vi "Measurement Loop.vi"(7 "measure call context in":refnum<class "Measure Call Context.lvclass">, 8 "error in":errorcluster, 9 "channel list":string, 10 "instrument handle":refnum<k15>, 11 "Measurement Configuration":T2={"Resource Name"="", "Measure Trigger Source"="", "Run Until"=6.0, "Current Limit"=0.01, "Voltage Level"=0.01, "Current Limit Range"=0.0, "Voltage Level Range"=5.0, "Aperture Time"=0.01666, "Current Unit"="mA", "Delimited Text"=","} {"Aperture Time" format="%#_6ps"; "Voltage Level Range" format="%#_6pV"; "Current Limit Range" format="%#_6pA"; "Voltage Level" format="%#_6pV"; "Current Limit" format="%#_6pA"; "Run Until" min=1.0 step=1.0 format="%#_g Samples"}) -> (0 "error out":errorcluster, 3 "Measurement Results":T1 {"Actual Aperture Time" format="%#_6ps"})   [LabVIEW 2025, in "DCPower Single Meas Per Trigger.lvclass"]
uses:
  DCPower Single Meas Per Trigger.lvclass
  DCPower Single Meas Per Trigger.lvclass/DCPower Single Meas Per Trigger.ctl
  Measurement Results.ctl
  <vilib>/Plug-In SDKs/Measurements/Measure Call Context/Measure Call Context.lvclass
  Measured Value.ctl
  <extravilib>/ChannelInstances/Stream-t'DCPower Single Meas Per Trigger.lvclass-Measured Value.ctl'.lvlib
  Measurement Configuration.ctl
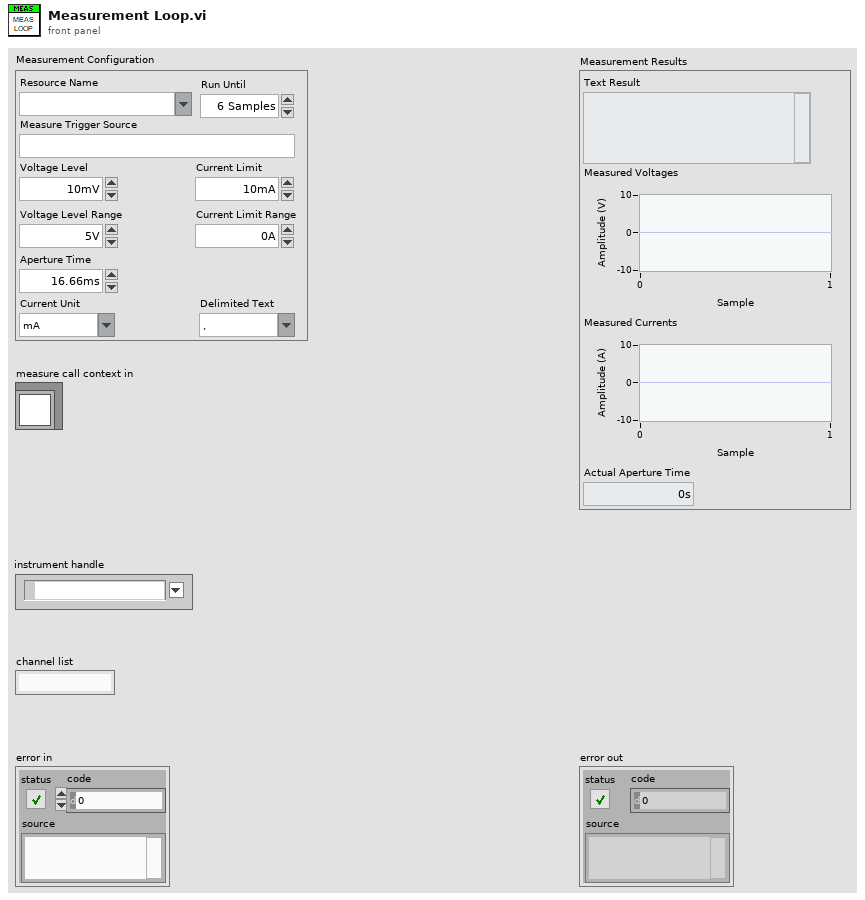
[diagram p1: front panel]
types:
  T1 = typedef "DCPower Single Meas Per Trigger.lvclass/Measurement Results.ctl" = cluster{"Text Result":string, "Measured Voltages":dbl[], "Measured Currents":dbl[], "Actual Aperture Time":dbl}
  T2 = typedef "DCPower Single Meas Per Trigger.lvclass/Measurement Configuration.ctl" = cluster{"Resource Name":string, "Measure Trigger Source":string, "Run Until":dbl, "Current Limit":dbl, "Voltage Level":dbl, "Current Limit Range":dbl, "Voltage Level Range":dbl, "Aperture Time":dbl, "Current Unit":string, "Delimited Text":string}
  T3 = typedef "DCPower Single Meas Per Trigger.lvclass/Measured Value.ctl" = cluster{"Voltages":dbl[], "Currents":dbl[], "In compliance":bool[]}
  T4 = typedef "Stream-t'DCPower Single Meas Per Trigger.lvclass-Measured Value.ctl'.lvlib/)Channel.ctl" = refnum<queue>
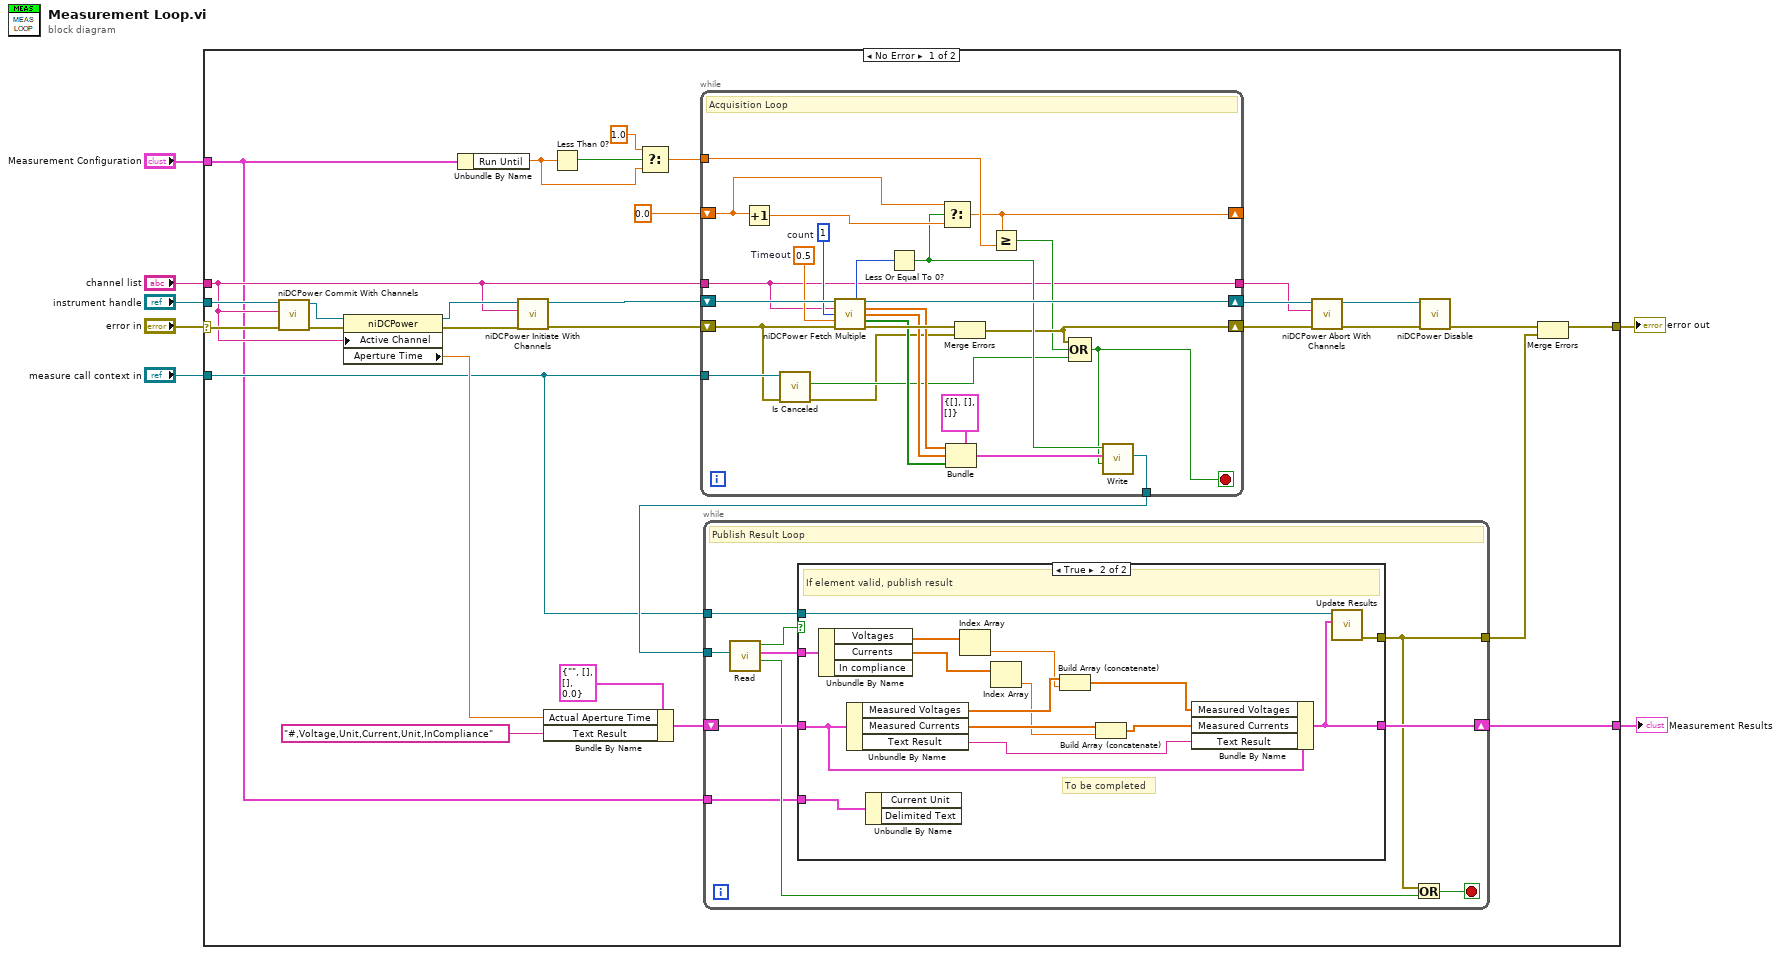
[diagram p0: block diagram]
diagram:
  n1 = case shown="No Error" "error in" {
    selector: "error in" -> [w34 w89]
    tunnel: "Measurement Configuration" -> [w8 _]
    tunnel: [w15 w89] -> w6
    tunnel: "instrument handle" -> [w30 _]
    tunnel: "channel list" -> [w28 _]
    tunnel: "measure call context in" -> [w16 _]
    tunnel: [w17 _] -> w1
    frame No Error {
      n2 = call <instrlib>:"niDCPower Commit With Channels.vi"("error in (no error)"=w34, "channel name"=w28, "instrument handle"=w30) -> ("error out"=w31:errorcluster, "instrument handle out"=w29:refnum<k15>)  [unwired: 7 in]
      n3 = property class="niDCPower"(reference=w29, error in=w31, "Active Channel"=w28) -> (reference out=w32:refnum<k15>, error out=w33:errorcluster, "Aperture Time"=w22:dbl)
      n4 = Unbundle By Name(w8) -> ("Run Until"=w24:dbl)
      n5 = call <instrlib>:"niDCPower Initiate With Channels.vi"("error in (no error)"=w33, "channel name"=w28, "instrument handle"=w32) -> ("error out"=w36:errorcluster, "instrument handle out"=w37:refnum<k15>)  [unwired: 7 in]
      n6 = Bundle By Name(cluster=T1 {"Text Result"="", "Measured Voltages"=[], "Measured Currents"=[], "Actual Aperture Time"=0.0} ("Measurement Results"), "Actual Aperture Time"=w22, "Text Result"="#,Voltage,Unit,Current,Unit,InCompliance") -> (w18:T1)
      n7 = Less Than 0?(x=w24) -> (x < 0?=w26:bool)
      n8 = Select(t=1.0, s=w26, f=w24) -> (s? t:f=w20:dbl)
      n9 = while {
        tunnel: w28 -> [w40]
        shift-right: [w61] -> w11
        shift-left: w37 -> [w62]
        shift-right: [w46] -> w35
        shift-left: w36 -> [w38]
        tunnel: w16 -> [w59]
        shift-right: [w44] -> _
        shift-left: 0.0 -> [w42]
        tunnel: w20 -> [w54]
        tunnel: [w48] -> w19
        tunnel: [w40] -> w10
        stop <- w39 stop-if-true
        w58 = 1  # count
        w60 = 0.5  # Timeout
        # "Acquisition Loop"
        n10 = Increment(x=w42) -> (x+1=w55:dbl)
        n11 = call <vilib>:"Is Canceled.vi"("error in"=w38, "measure call context in"=w59) -> ("error out"=w45:errorcluster, "is canceled?"=w47:bool)  [unwired: 7 in, 1 out]
        n12 = call <instrlib>:"niDCPower Fetch Multiple.vi"("instrument handle"=w62, "channel name"=w40, "count (1)"=w58, "timeout (1.0)"=w60, "error in (no error)"=w38) -> ("actual count"=w56:i32, "instrument handle out"=w61:refnum<k15>, "voltage measurements"=w53:dbl[], "current measurements"=w52:dbl[], "in compliance"=w51:bool[], "error out"=w57:errorcluster)  [unwired: 5 in]
        n13 = Less Or Equal To 0?(x=w56) -> (x <= 0?=w49:bool)
        n14 = Select(t=w42, s=w49, f=w55) -> (s? t:f=w44:dbl)
        n15 = Bundle(cluster=T3 {"Voltages"=[], "Currents"=[], "In compliance"=[]} ("output cluster"), "Voltages"=w53, "Currents"=w52, "In compliance"=w51) -> (w41:T3)
        n16 = Merge Errors(w57, w45) -> (w46:errorcluster)
        n17 = Greater Or Equal?(x=w44, y=w54) -> (x >= y?=w43:bool)
        n18 = Compound Arithmetic op=OR(w46, w43, w47) -> (w39:bool)
        n19 = call <extravilib>:"Write.vi"("last element? (F)"=w39, "element"=w41, "element valid? (T)"=w49) -> ("channel"=w48:T4)  [unwired: 6 in, 2 out]
      }
      n20 = while {
        shift-right: [w72] -> w17
        shift-left: w18 -> [w68]
        tunnel: w19 -> [w71]
        tunnel: w16 -> [w66]
        tunnel: [w64] -> w14
        tunnel: w8 -> [w63]
        stop <- w65 stop-if-true
        # "Publish Result Loop"
        n21 = call <extravilib>:"Read.vi"("channel"=w71) -> ("last element?"=w67:bool, "element"=w70:T3, "element valid?"=w69:bool)  [unwired: 6 in, 2 out]
        n22 = case shown="True" w69 {
          tunnel: [w73 w77] -> w72
          tunnel: w70 -> [_ w88]
          tunnel: w68 -> [w73 w86]
          tunnel: w66 -> [_ w78]
          tunnel: [_ w76] -> w64
          tunnel: w63 -> [_ w74]
          frame False {
          }
          frame True {
            # "To be completed"
            # "If element valid, publish result"
            n23 = Unbundle By Name(w88) -> ("Voltages"=w87:dbl[], "Currents"=w83:dbl[])  [unwired: 1 out]
            n24 = Unbundle By Name(w86) -> ("Measured Voltages"=w85:dbl[], "Measured Currents"=w81:dbl[], "Text Result"=w75:string)
            n25 = Unbundle By Name(w74) -> ()  [unwired: 2 out]
            n26 = Index Array(array=w87) -> (element=w84:dbl)  [unwired: 1 in]
            n27 = Index Array(array=w83) -> (element=w80:dbl)  [unwired: 1 in]
            n28 = Build Array (concatenate)(w85, w84) -> (w82:dbl[])
            n29 = Build Array (concatenate)(w81, w80) -> (w79:dbl[])
            n30 = Bundle By Name(cluster=w86, "Measured Voltages"=w82, "Measured Currents"=w79, "Text Result"=w75) -> (w77:T1)
            n31 = call <vilib>:"Update Results.vi"("measurement results"=w77, "measure call context in"=w78) -> ("error out"=w76:errorcluster)  [unwired: 8 in, 1 out]
          }
        }
        n32 = Or(x=w64, y=w67) -> (x .or. y?=w65:bool)
      }
      n33 = call <instrlib>:"niDCPower Abort With Channels.vi"("error in (no error)"=w35, "channel name"=w10, "instrument handle"=w11) -> ("error out"=w12:errorcluster, "instrument handle out"=w9:refnum<k15>)  [unwired: 7 in]
      n34 = call <instrlib>:"niDCPower Disable.vi"("error in (no error)"=w12, "instrument handle"=w9) -> ("error out"=w13:errorcluster)  [unwired: 8 in, 1 out]
      n35 = Merge Errors(w13, w14) -> (w15:errorcluster)
    }
    frame Error {
    }
  }
  "Measurement Results" <- w1
  "error out" <- w6
